vi "FunctDataMgr.Read Result State.vi"(8 "error in (no error)":errorcluster, 11 "FunctDataMgr in":refnum<class "FunctDataMgr.lvclass">) -> (0 "error out":errorcluster, 2 "Result Info":T1={"State"=enum."Passing", "Code"=0, "Description"=""}, 3 "FunctDataMgr out":refnum<class "FunctDataMgr.lvclass">)   [LabVIEW 2018, in "FunctDataMgr.lvclass"]
uses:
  FunctDataMgr.lvclass
  <vilib>/KATE/SeqMgr/SeqMgr.Result Info.ctl
  <vilib>/KATE/SeqMgr/SeqMgr.Result State Enum.ctl
  FunctDataMgr.lvclass/FunctDataMgr.ctl
  <vilib>/KATE/SeqMgr/SeqMgr.lvlib
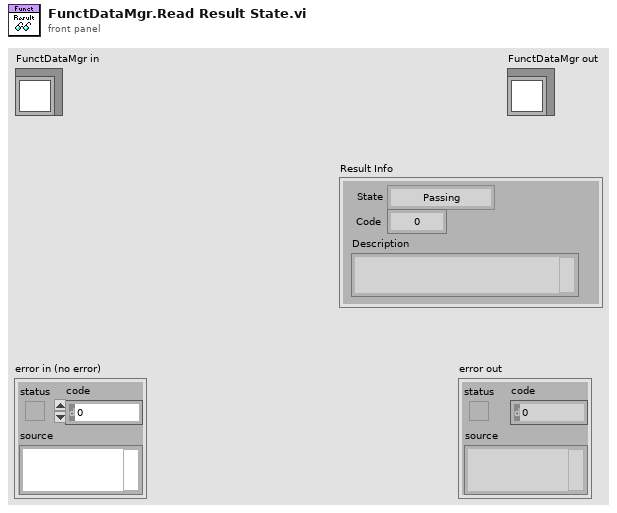
[diagram p1: front panel]
types:
  T1 = typedef "KATE_Lib.lvlib/SeqMgr.lvlib/SeqMgr.Result Info.ctl" = cluster{"State":T2, "Code":i32, "Description":string}
  T2 = typedef "KATE_Lib.lvlib/SeqMgr.lvlib/SeqMgr.Result State Enum.ctl" = enum16{"None", "Passing", "Failing", "PASS", "FAIL", "ABORT", "ERROR"}
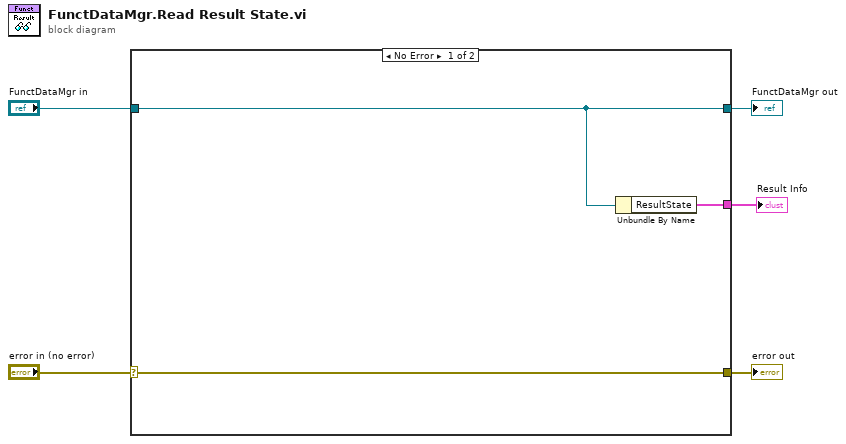
[diagram p0: block diagram]
diagram:
  n1 = case shown="No Error" "error in (no error)" {
    selector: "error in (no error)" -> [w8 w10]
    tunnel: [w8 w10] -> w4
    tunnel: [w7 w9] -> w2
    tunnel: "FunctDataMgr in" -> [w7 w9]
    tunnel: [w6 _] -> w1
    frame No Error {
      n2 = Unbundle By Name(w7) -> ("ResultState"=w6:T1)
    }
    frame Error {
    }
  }
  "error out" <- w4
  "FunctDataMgr out" <- w2
  "Result Info" <- w1
